vi "PXIUI.vi"() -> ()   [LabVIEW 2013, in "PLTarget PXI.lvclass"]
uses:
  PLTarget PXI.lvclass
  <vilib>/NI/Configuration Framework/Node/NodeRef.ctl
  <vilib>/NI/Configuration Framework/Node/NISE_CEF_Node.lvclass
  <vilib>/NI/AMC/Message Queue.ctl
  <vilib>/NI/AMC/Message.ctl
  <vilib>/NI/Tools/Keyed Array/KeyedArray.ctl
  <vilib>/NI/Configuration Framework/Node/UserEventRef.ctl
  <vilib>/NI/Configuration Framework/Controls/EventCluster.ctl
  <vilib>/NI/Tag Bus Module Framework/root configuration/Target Types.ctl
  <vilib>/NI/Configuration Framework/Node/RefreshUIEvent.ctl
  <vilib>/NI/Configuration Framework/Node/CacheState.ctl
  <vilib>/NI/Configuration Framework/Node/StopEvent.ctl
  <vilib>/NI/Configuration Framework/Node/NodeChangeEvent.ctl
  Configuration Editor/subVIs/Additional Files Array.ctl
  Configuration Editor/Classes/TBM Configuration Node/deployment configuration.ctl
  <vilib>/Utility/miscctls.llb/LVPositionTypeDef.ctl
  PLTarget PXI.lvclass/PLTarget PXI.ctl
  Framework Configuration Classes/target configuration/PL_Target Configuration.lvclass/PL_Target Configuration.ctl
  Configuration Editor/Classes/Targets/Targets.lvclass/Targets.ctl
  <vilib>/NI/Configuration Framework/serializable node/NISE_CEF_serializable node.lvclass
  <vilib>/NI/Tag Bus Module Framework/root configuration/TBM configuration.lvclass
  Configuration Editor/Classes/Targets/Write additional files.vi
  Configuration Editor/Classes/Targets/Read additional files.vi
  <vilib>/NI/Configuration Framework/serializable configuration/set alias.vi
  <vilib>/NI/Configuration Framework/serializable configuration/get alias.vi
  <vilib>/NI/Configuration Framework/serializable configuration/NISE_CEF_serializable configuration.lvclass
  Framework Configuration Classes/target configuration/PL_Target Configuration.lvclass
  Configuration Editor/Classes/Targets/Targets.lvclass
  <vilib>/NI/DCAF UI Toolkit/Controls/DCAF UI Elements.lvlib
  <vilib>/NI/Tools/Keyed Array/Tools_KeyedArray.lvlib
  <vilib>/NI/AMC/AMC.lvlib
  <vilib>/NI/Configuration Framework/NISE_CEF_TreeControl.lvlib
  Configuration Editor/Classes/TBM Configuration Node/TBM Configuration Node.lvclass
panel:
  in  "Top Level Tab Control":enum32{"Configuration", "Additional Files"}(tab)
  in  "Target Type":T1=enum."Pharlap"
  in  "IP":string
  in  "Name":string
  in  "Includes file path":path
  in  "path to deploy on target relative to root (c:\\ or /home/lvuser/)":path
  in  "generate includes file":bool
  in  "Additional Files":T2
  in  "node change":T4
  in  "stop event":T5
  in  "cache state":T6
  in  "refresh UI":T7
  in  "open fp?":bool=TRUE
  in  "user event":T8
  in  "main queue":T9
  in  "node ref":T10
  # "Target Information"
  # "Deployment Settings"
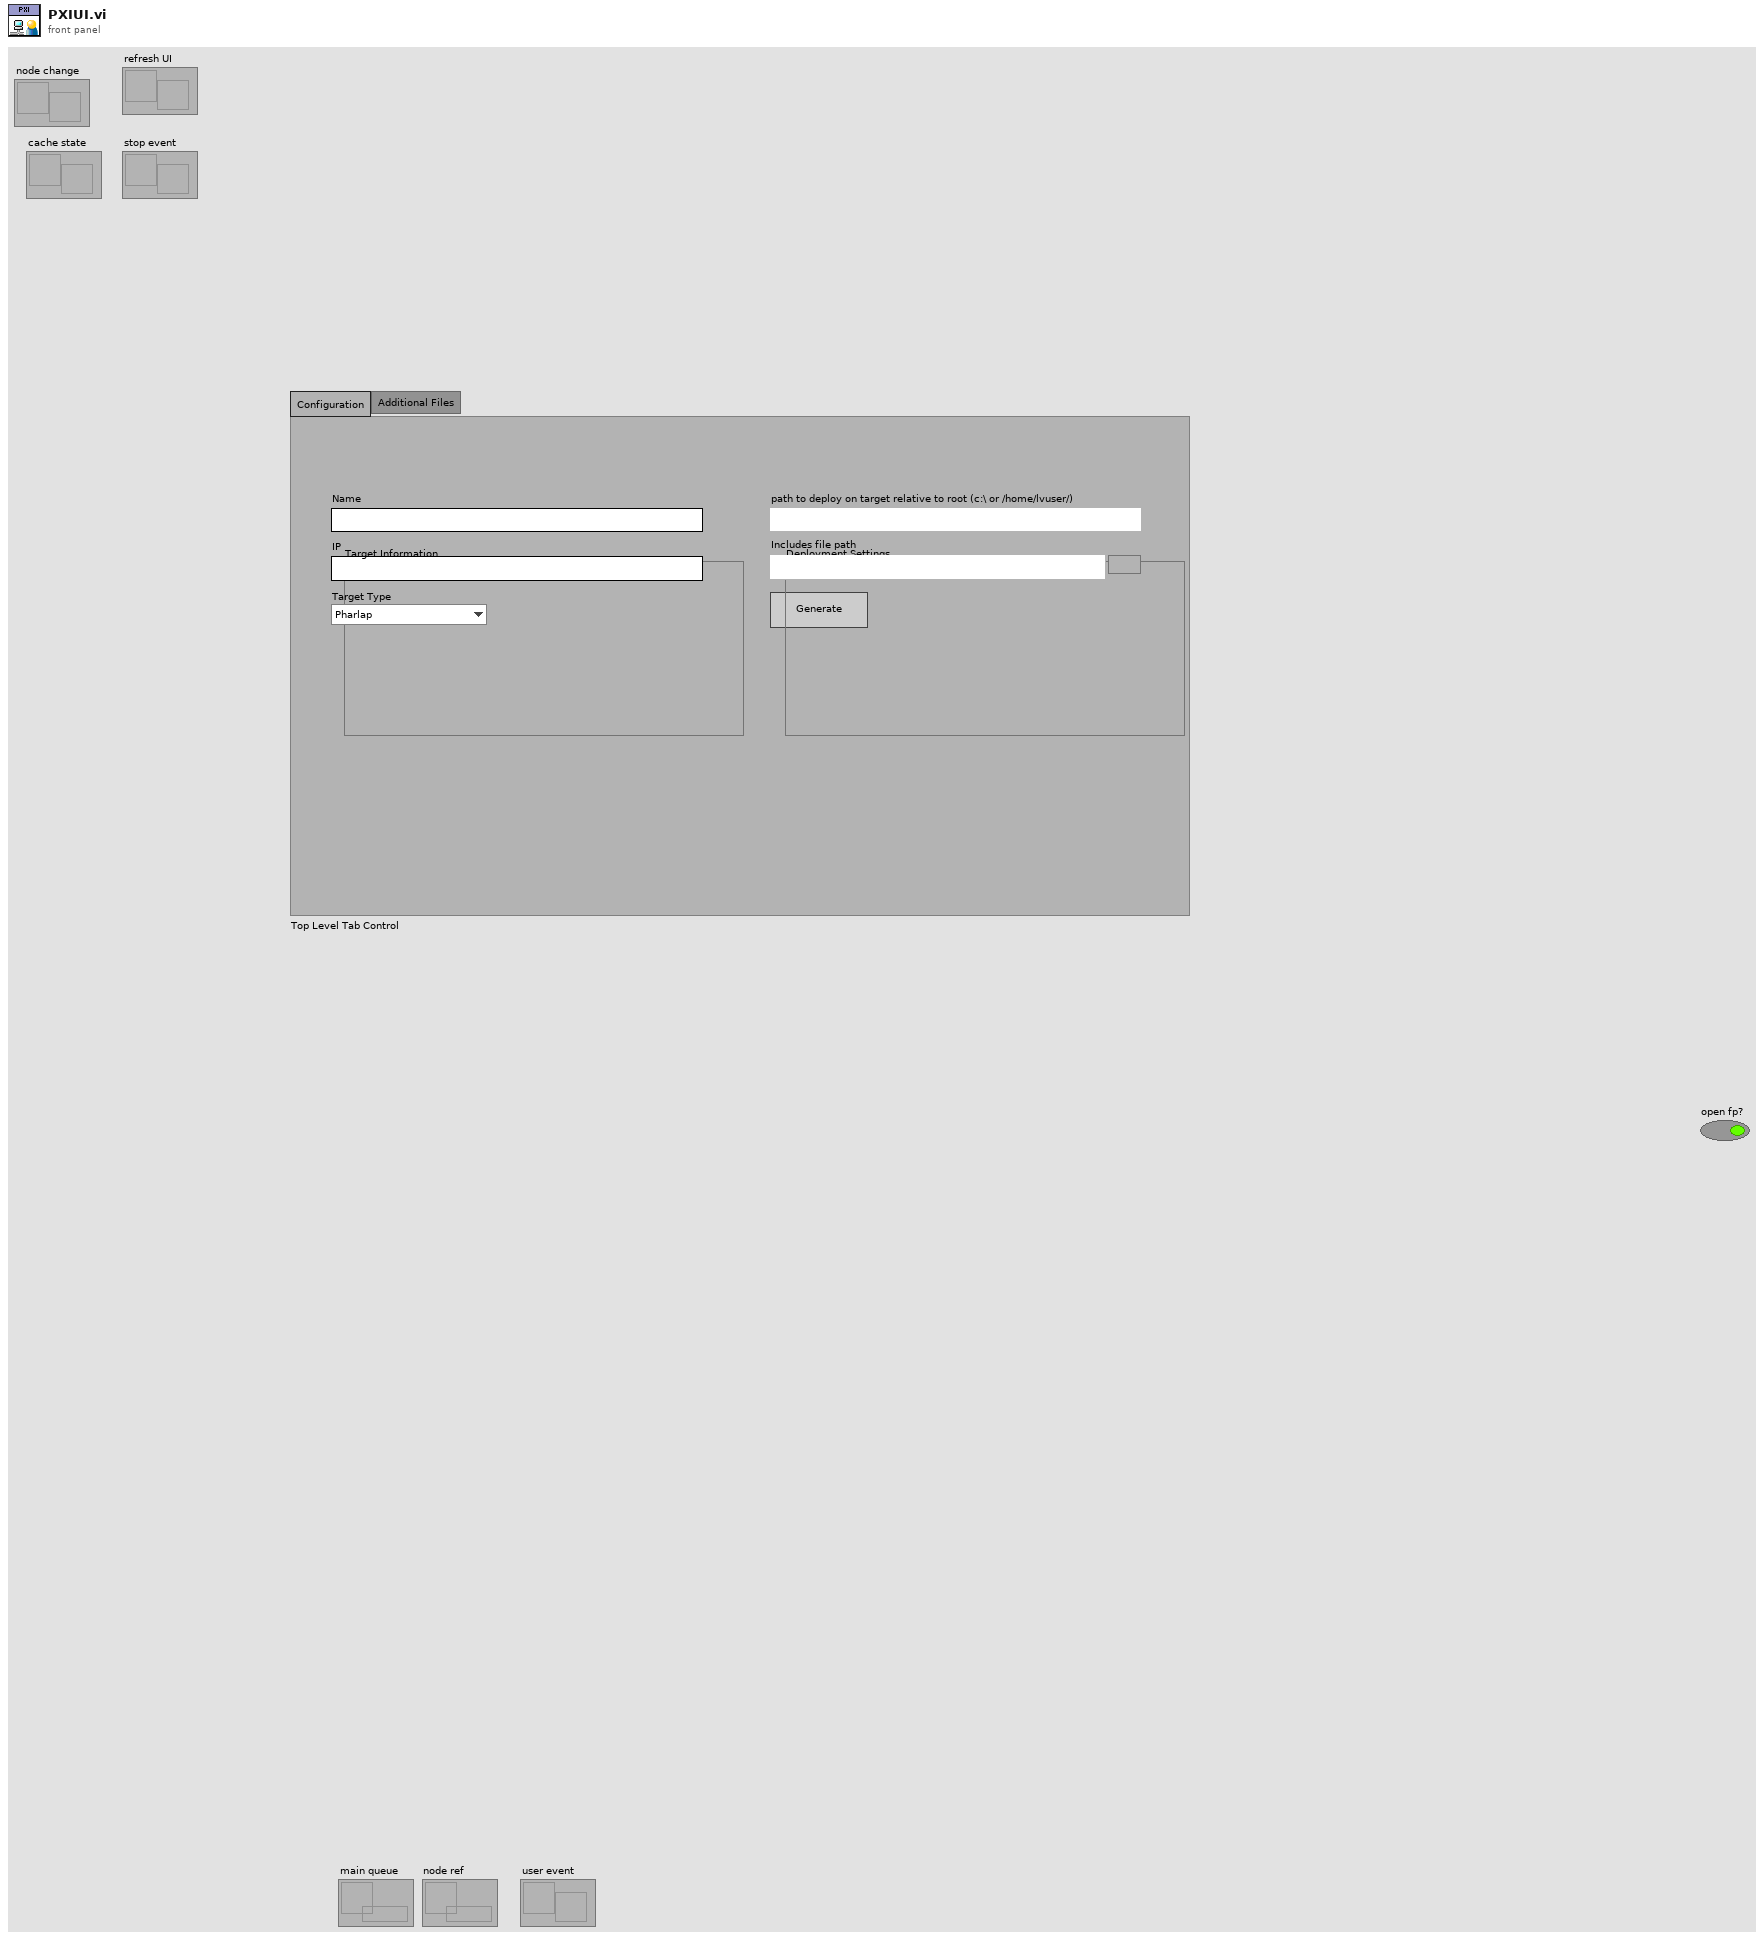
[diagram p1: front panel]
types:
  T1 = typedef "TBM configuration.lvclass/Target Types.ctl" = enum16{"Windows", "Mac", "Linux", "Linux RT ARM", "VxWorks", "Pharlap", "Other", "Linux RT x64"}
  T2 = typedef "Additional Files Array.ctl" = T3[]
  T3 = typedef "PL Framework Configuration Tool.lvlib/TBM Configuration Node.lvclass/deployment configuration.ctl" = cluster{"local path":path, "remote path (relative to root)":path}
  T4 = typedef "NISE_CEF_Node.lvclass/NodeChangeEvent.ctl" = refnum<user-event>
  T5 = typedef "NISE_CEF_Node.lvclass/StopEvent.ctl" = refnum<user-event>
  T6 = typedef "NISE_CEF_Node.lvclass/CacheState.ctl" = refnum<user-event>
  T7 = typedef "NISE_CEF_Node.lvclass/RefreshUIEvent.ctl" = refnum<user-event>
  T8 = typedef "NISE_CEF_Node.lvclass/UserEventRef.ctl" = refnum<user-event>
  T9 = typedef "AMC.lvlib/Message Queue.ctl" = refnum<queue>
  T10 = typedef "NISE_CEF_Node.lvclass/NodeRef.ctl" = refnum<data-value>
  T11 = typedef "LVPositionTypeDef.ctl" = cluster{"Left":i32, "Top":i32}
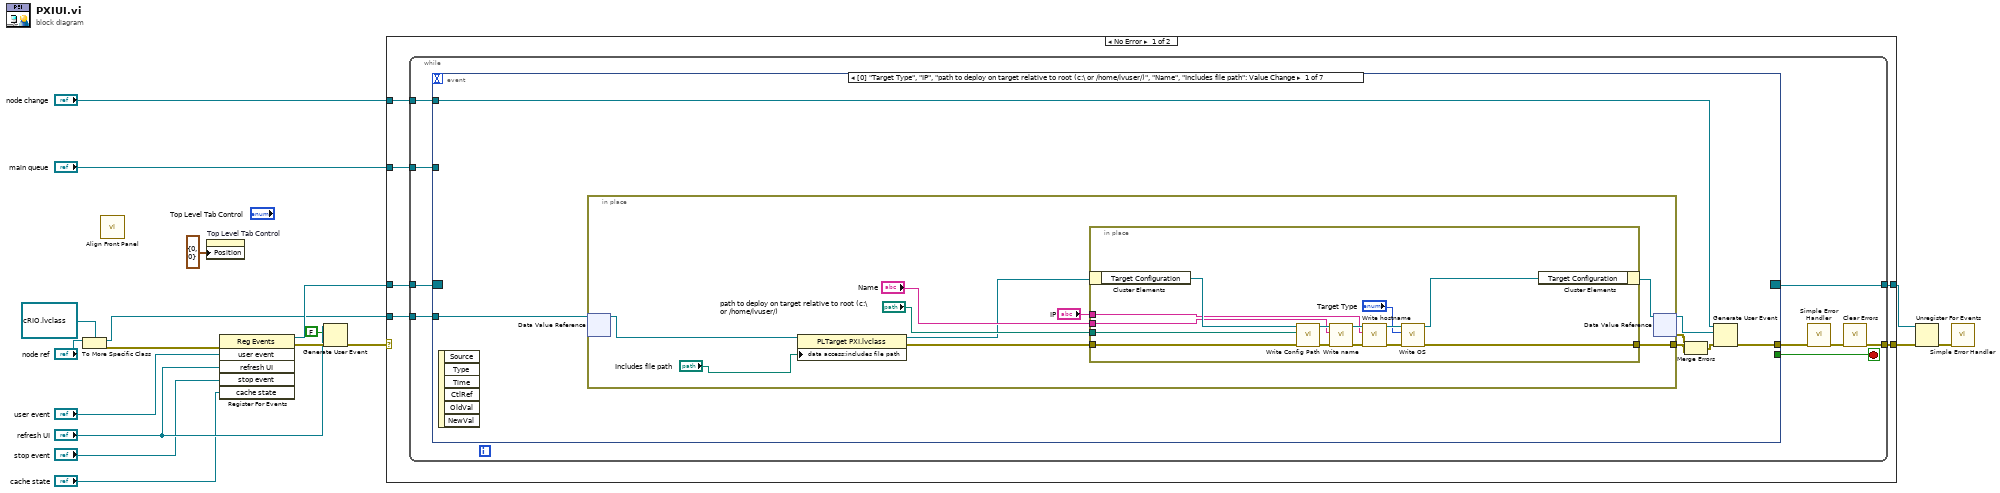
[diagram p0: block diagram]
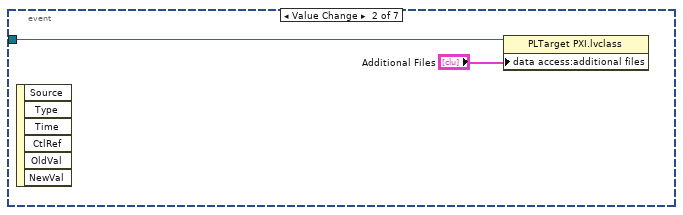
[diagram p2: hidden frame]
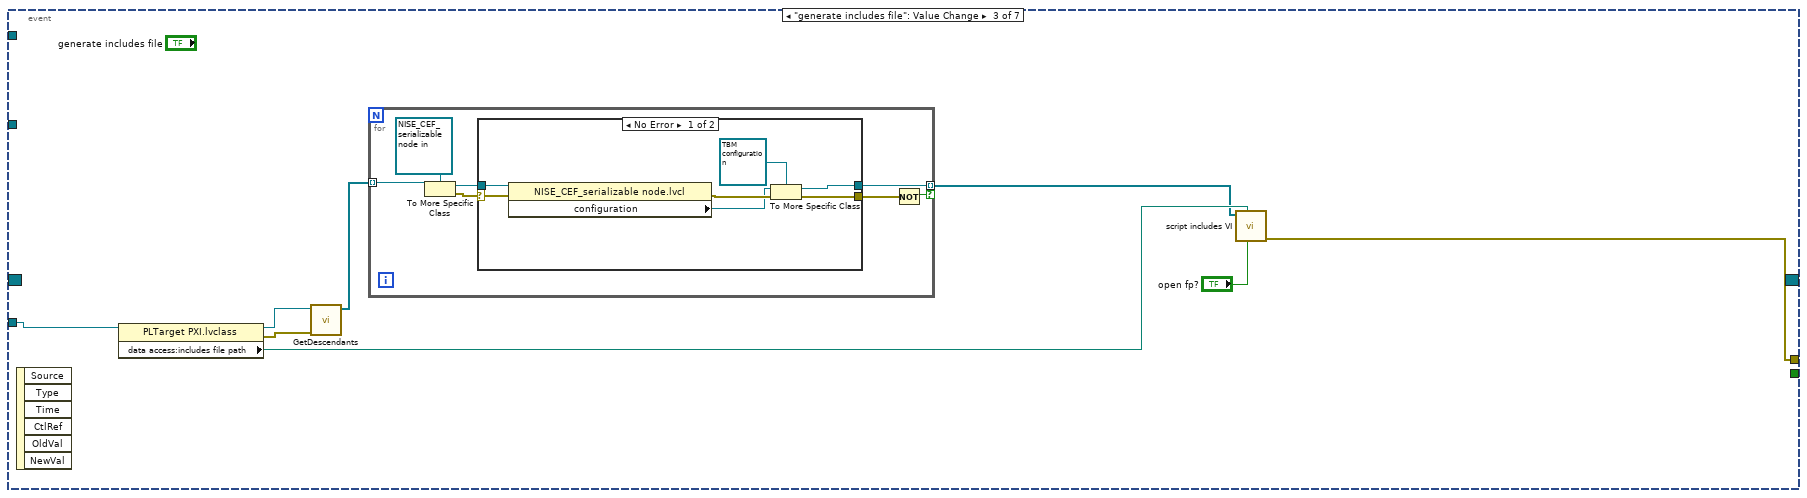
[diagram p3: hidden frame]
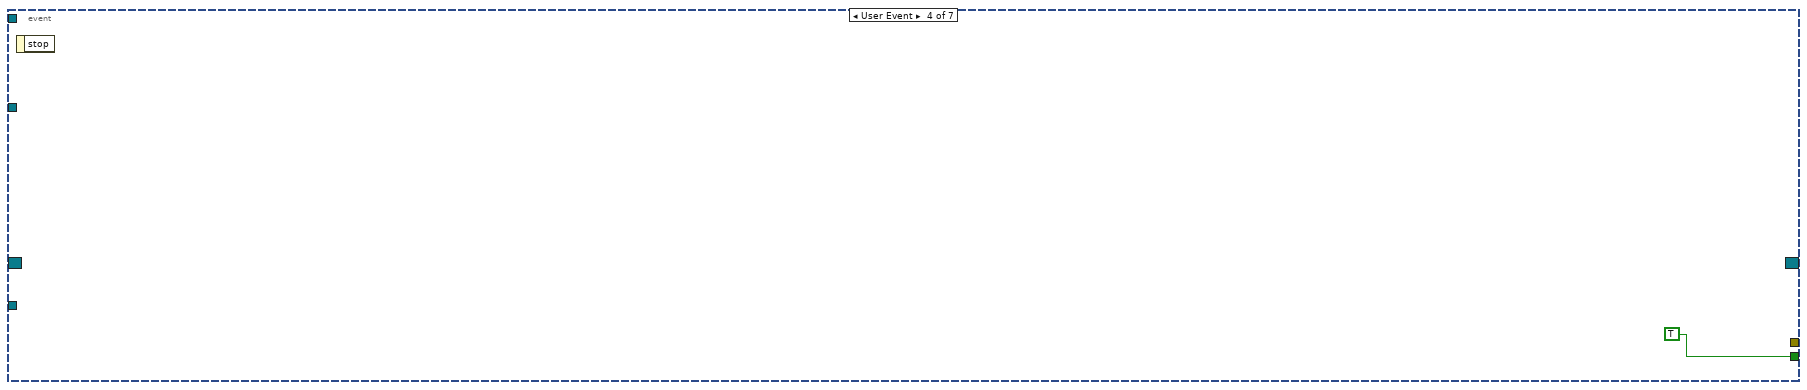
[diagram p5: hidden frame]
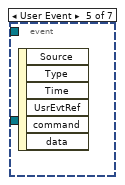
[diagram p6: hidden frame]
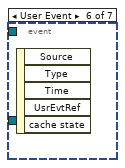
[diagram p7: hidden frame]
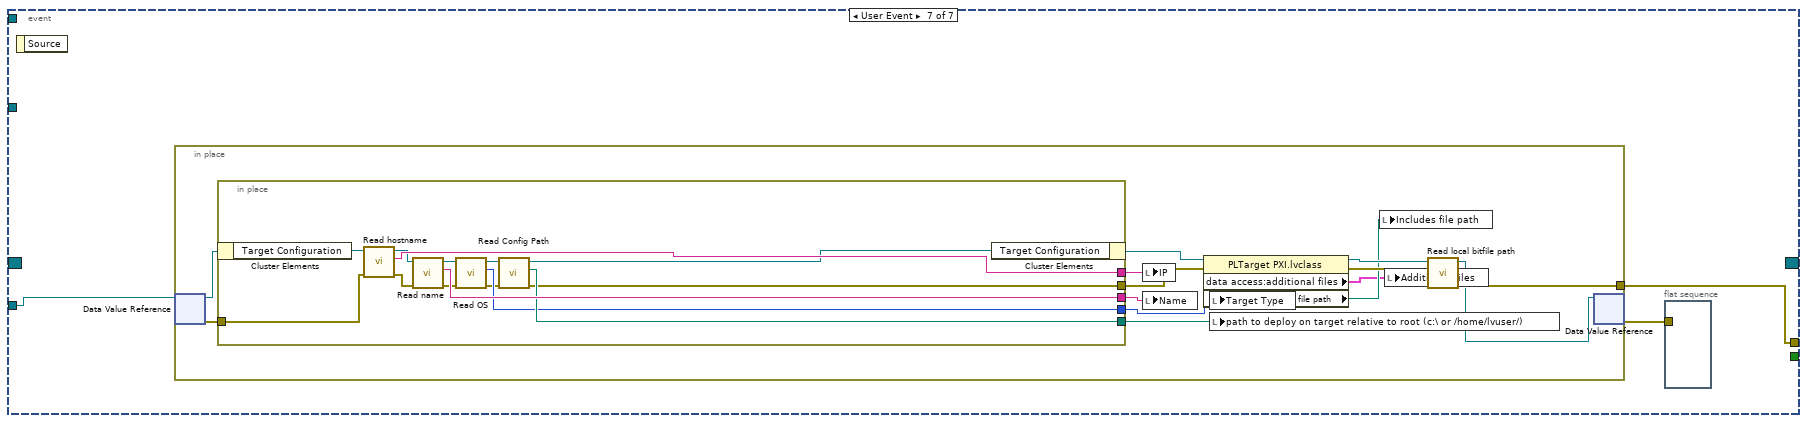
[diagram p8: hidden frame]
diagram:
  n1 = To More Specific Class(target class=refnum<data-value> refnum ("data value reference"), reference="node ref") -> (specific class reference=w5:refnum<data-value>, error out=w6:errorcluster)  [unwired: 1 in]
  n2 = call <vilib>:"Align Front Panel.vi"() -> ()  [unwired: 10 in, 2 out]
  n3 = property on="Top Level Tab Control" class="TabCtl (strict)"("Position"=T11 {"Left"=0, "Top"=0}) -> ()  [unwired: 2 in, 2 out]
  n4 = register-events(error in=w6, "user event", "refresh UI", "stop event", "cache state") -> (reference out=w16:refnum<event-registration>, error out=w13:errorcluster)  [unwired: 1 in]
  n5 = Generate User Event(user event="refresh UI", event data cluster=FALSE ("event data"), error in=w13) -> (error out=w7:errorcluster)  [unwired: 1 in, 1 out]
  n6 = case shown="No Error" w7 {
    selector: w7 -> [_ w121]
    tunnel: w5 -> [w24 _]
    tunnel: "main queue" -> [w23 _]
    tunnel: w16 -> [w22 w122]
    tunnel: [w21 w122] -> w15
    tunnel: [w20 w121] -> w14
    tunnel: "node change" -> [w19 _]
    frame No Error {
      n7 = while {
        tunnel: w24 -> [w33]
        tunnel: w23 -> [w32]
        tunnel: w22 -> [w31]
        tunnel: [w30] -> w21
        tunnel: [w26] -> w20
        tunnel: w19 -> [w25]
        stop <- w29 stop-if-true
        n8 = event shown="[0] \"Target Type\", \"IP\", \"path to deploy on target relative to root (c:\\ or /home/lvuser/)\", \"Name\", \"Includes file path\": Value Change" {
          selector: w31 -> [_ _ _ _ _ _ _]
          dyn-events: [_ _ _ _ _ _ _] -> w30
          timeout: _ -> [_ _ _ _ _ _ _]
          tunnel: w33 -> [w40 w65 w73 _ _ _ w92]
          tunnel: w32 -> [_ _ _ _ _ _ _]
          tunnel: [_ _ _ TRUE _ _ _] -> w29
          tunnel: [w38 _ w70 _ _ _ w91] -> w28
          tunnel: w25 -> [w37 _ _ _ _ _ _]
          event "IP", "path to deploy on target relative to root (c:\\ or /home/lvuser/)", "Name", "Includes file path": Value Change {
            n9 = event-data() -> ()  [unwired: 1 in, 6 out]
            n10 = in-place {
              in-place-border: [w45] -> w39
              n11 = in-place-dvr #1(w40) -> (w44:refnum<class "PLTarget PXI.lvclass">)  [unwired: 1 out]
              n12 = property class="PLTarget PXI.lvclass"(reference=w44, "data access:includes file path"="Includes file path") -> (reference out=w42:refnum<class "PLTarget PXI.lvclass">, error out=w43:errorcluster)  [unwired: 1 in]
              n13 = in-place {
                in-place-border: "path to deploy on target relative to root (c:\\ or /home/lvuser/)" -> [w62]
                in-place-border: "IP" -> [w59]
                in-place-border: "Name" -> [w58]
                in-place-border: w43 -> [w52]
                in-place-border: [w51] -> w45
                n14 = in-place-cluster #2(w42) -> ("Target Configuration"=w63:refnum<class "PL_Target Configuration.lvclass">)
                n15 = call "Write Config Path.vi"("error in"=w52, "Config Path"=w62, "PL_Local Target Configuration in"=w63) -> ("error out"=w55:errorcluster, "PL_Local Target Configuration out"=w61:refnum<class "PL_Target Configuration.lvclass">)  [unwired: 7 in]
                n16 = call "Write name.vi"("error in"=w55, "name"=w58, "PL_Local Target Configuration in"=w61) -> ("error out"=w54:errorcluster, "PL_Local Target Configuration out"=w60:refnum<class "PL_Target Configuration.lvclass">)  [unwired: 7 in]
                n17 = call "Write hostname.vi"("error in"=w54, "hostname"=w59, "PL_Target Configuration in"=w60) -> ("error out"=w53:errorcluster, "PL_Target Configuration out"=w57:refnum<class "PL_Target Configuration.lvclass">)  [unwired: 7 in]
                n18 = call "Write OS.vi"("error in"=w53, "Target Types"="Target Type", "PL_Target Configuration in"=w57) -> ("error out"=w51:errorcluster, "PL_Target Configuration out"=w50:refnum<class "PL_Target Configuration.lvclass">)  [unwired: 7 in]
                n19 = in-place-cluster #2("Target Configuration"=w50) -> (w49:refnum<class "PLTarget PXI.lvclass">)
              }
              n20 = in-place-dvr #1(w49) -> (w36:refnum<data-value>, w34:errorcluster)
            }
            n21 = Merge Errors(w39, w34) -> (w35:errorcluster)
            n22 = Generate User Event(user event=w37, event data cluster=w36, error in=w35) -> (error out=w38:errorcluster)  [unwired: 1 in, 1 out]
          }
          event Value Change {
            n23 = event-data() -> ()  [unwired: 1 in, 6 out]
            n24 = property class="PLTarget PXI.lvclass"(reference=w65, "data access:additional files"="Additional Files") -> ()  [unwired: 1 in, 2 out]
          }
          event "generate includes file": Value Change {
            n25 = event-data() -> ()  [unwired: 1 in, 6 out]
            n26 = property class="PLTarget PXI.lvclass"(reference=w73) -> (reference out=w68:refnum<data-value>, error out=w69:errorcluster, "data access:includes file path"=w71:path)  [unwired: 1 in]
            n27 = call <vilib>:"GetDescendants.vi"("error in"=w69, "node in"=w68) -> ("descendants"=w67:refnum<data-value>[])  [unwired: 8 in, 1 out]
            n28 = for {
              tunnel: w67 -> [w80] mode=indexing
              tunnel: [w76] -> w66 mode=indexing if=w74
              n29 = To More Specific Class(target class=refnum<data-value> refnum, reference=w80) -> (specific class reference=w77:refnum<data-value>, error out=w78:errorcluster)  [unwired: 1 in]
              n30 = case shown="No Error" w78 {
                selector: w78 -> [w86 w88]
                tunnel: w77 -> [w87 _]
                tunnel: [w81 _] -> w76
                tunnel: [w84 w88] -> w75
                frame No Error {
                  n31 = property class="NISE_CEF_serializable node.lvcl"(reference=w87, error in=w86) -> (error out=w85:errorcluster, "configuration"=w83:refnum<class "NISE_CEF_serializable configuration.lvclass">)  [unwired: 1 out]
                  n32 = To More Specific Class(target class=refnum<class "TBM configuration.lvclass"> refnum ("configuration"), reference=w83, error in=w85) -> (specific class reference=w81:refnum<class "TBM configuration.lvclass">, error out=w84:errorcluster)
                }
                frame Error {
                }
              }
              n33 = Not(x=w75) -> (.not. x?=w74:bool)
            }
            n34 = call "script includes VI.vi"("open fp?"="open fp?", "vi path (blank=new)"=w71, "cfg objects"=w66) -> ("error out"=w70:errorcluster)  [unwired: 8 in]
          }
          event User Event {
            n35 = event-data() -> ()  [unwired: 1 in, 1 out]
          }
          event User Event {
            n36 = event-data() -> ()  [unwired: 1 in, 6 out]
          }
          event User Event {
            n37 = event-data() -> ()  [unwired: 1 in, 5 out]
          }
          event User Event {
            n38 = event-data() -> ()  [unwired: 1 in, 1 out]
            n39 = in-place {
              in-place-border: [w99] -> w91
              n40 = in-place-dvr #3(w92) -> (w103:refnum<class "PLTarget PXI.lvclass">, w101:errorcluster)
              n41 = in-place {
                in-place-border: [w120] -> w106
                in-place-border: [w115] -> w104
                in-place-border: [w119] -> w105
                in-place-border: [w113] -> w102
                in-place-border: w101 -> [w109]
                in-place-border: [w108] -> w100
                n42 = in-place-cluster #4(w103) -> ("Target Configuration"=w116:refnum<class "PL_Target Configuration.lvclass">)
                n43 = call "Read hostname.vi"("error in"=w109, "PL_Target Configuration in"=w116) -> ("error out"=w112:errorcluster, "hostname"=w119:string, "PL_Target Configuration out"=w117:refnum<class "PL_Target Configuration.lvclass">)  [unwired: 7 in]
                n44 = call "Read name.vi"("error in"=w112, "PL_Local Target Configuration in"=w117) -> ("error out"=w111:errorcluster, "name"=w120:string, "PL_Local Target Configuration out"=w118:refnum<class "PL_Target Configuration.lvclass">)  [unwired: 7 in]
                n45 = call "Read OS.vi"("error in"=w111, "PL_Target Configuration in"=w118) -> ("error out"=w110:errorcluster, "Target Types"=w113:T1, "PL_Target Configuration out"=w114:refnum<class "PL_Target Configuration.lvclass">)  [unwired: 7 in]
                n46 = call "Read Config Path.vi"("error in"=w110, "PL_Local Target Configuration in"=w114) -> ("error out"=w108:errorcluster, "Config Path"=w115:path, "PL_Local Target Configuration out"=w107:refnum<class "PL_Target Configuration.lvclass">)  [unwired: 7 in]
                n47 = in-place-cluster #4("Target Configuration"=w107) -> (w96:refnum<class "PLTarget PXI.lvclass">)
              }
              n48 = local write "IP"(w105) -> ()
              n49 = local write "Name"(w106) -> ()
              n50 = property class="PLTarget PXI.lvclass"(reference=w96, error in=w100) -> (reference out=w95:refnum<class "PLTarget PXI.lvclass">, error out=w97:errorcluster, "data access:additional files"=w93:T3[], "data access:includes file path"=w94:path)
              n51 = local write "Target Type"(w102) -> ()
              n52 = local write "path to deploy on target relative to root (c:\\ or /home/lvuser/)"(w104) -> ()
              n53 = local write "Includes file path"(w94) -> ()
              n54 = local write "Additional Files"(w93) -> ()
              n55 = call "Read local bitfile path.vi"("error in"=w97, "Targets in"=w95) -> ("error out"=w99:errorcluster, "Targets out"=w98:refnum<class "PLTarget PXI.lvclass">)  [unwired: 7 in, 1 out]
              n56 = in-place-dvr #3(w98) -> (w90:errorcluster)  [unwired: 1 out]
            }
            n57 = flat-sequence {
              tunnel: w90 -> [_]
              frame #0 {
              }
            }
          }
        }
        n58 = call <vilib>:"Simple Error Handler.vi"("error in (no error)"=w28) -> ("error out"=w27:errorcluster)  [unwired: 4 in, 4 out]
        n59 = call <vilib>:"Clear Errors.vi"("error in (no error)"=w27) -> ("error out"=w26:errorcluster)  [unwired: 6 in]
      }
    }
    frame Error {
    }
  }
  n60 = Unregister For Events(event registration refnum=w15, error in=w14) -> (error out=w4:errorcluster)
  n61 = call <vilib>:"Simple Error Handler.vi"("error in (no error)"=w4) -> ()  [unwired: 4 in, 5 out]
